vi "route_Ver.2.0.vi"(8 "error in (no error)":errorcluster, 9 "Position":T2, 11 "?":T1) -> (0 "error out":errorcluster, 1 "Position out":T2)   [LabVIEW 2019]
uses:
  subVI/move/position cluster.ctl
  route_name.ctl
  subVI/move control/move and align/move_cluster.ctl
  align position.ctl
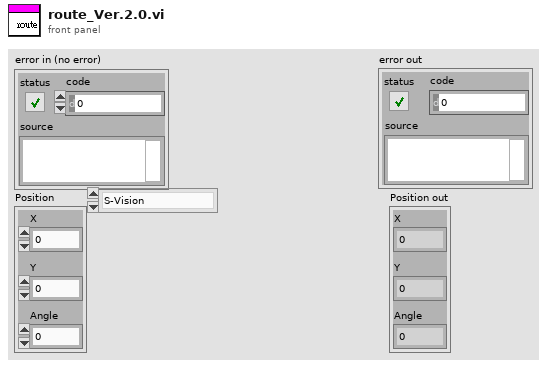
[diagram p1: front panel]
types:
  T1 = typedef "route_name.ctl" = enum16{"S-Vision", "Vision-R1", "Vision-R2", "Vision-R3", "Vision-R4", "Vision-R5", "R1-Vision", "R2-Vision", "R3-Vision", "R4-Vision", "R5-Vision", "Vision-box", "box-recycle", "recycle-box", "box-Vision", "Vision-S", "R2-R3"}
  T2 = typedef "position cluster.ctl" = cluster{"X":dbl, "Y":dbl, "Angle":dbl}
  T3 = typedef "move_cluster.ctl" = cluster{"X":dbl, "Y":dbl, "degree":dbl, "speed":dbl}
  T4 = typedef "align position.ctl" = enum16{"S align", "vision align", "box align", "box to room align"}
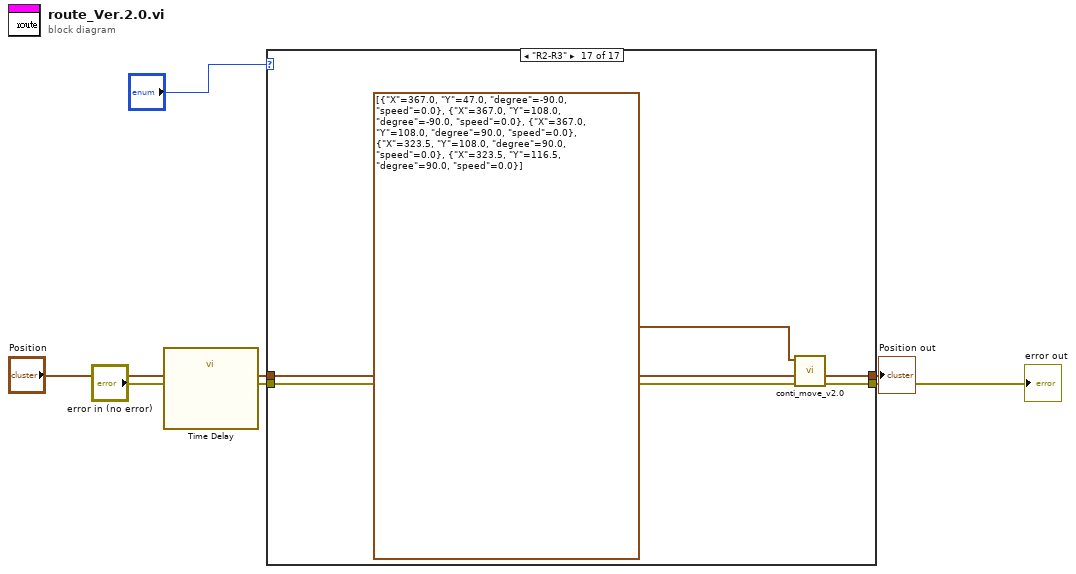
[diagram p0: block diagram]
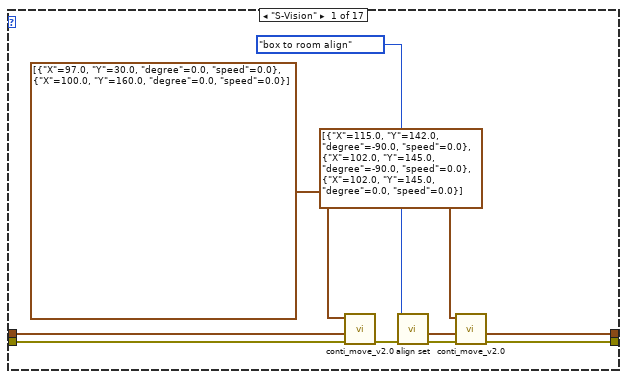
[diagram p2: hidden frame]
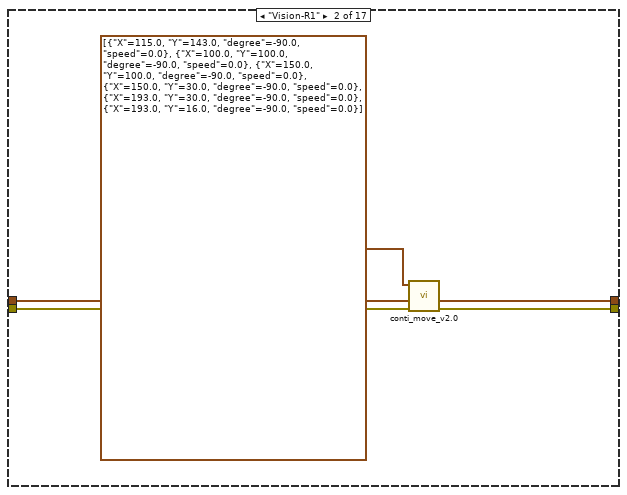
[diagram p3: hidden frame]
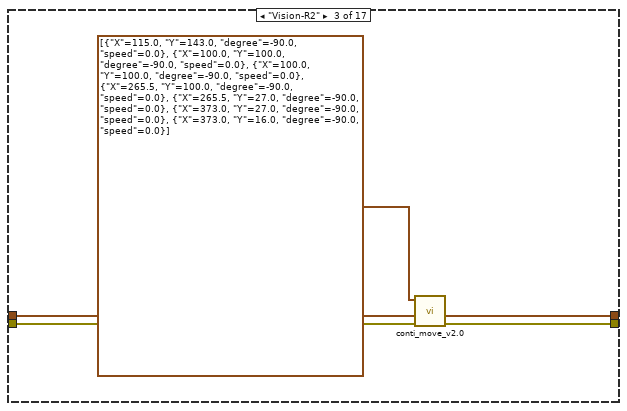
[diagram p4: hidden frame]
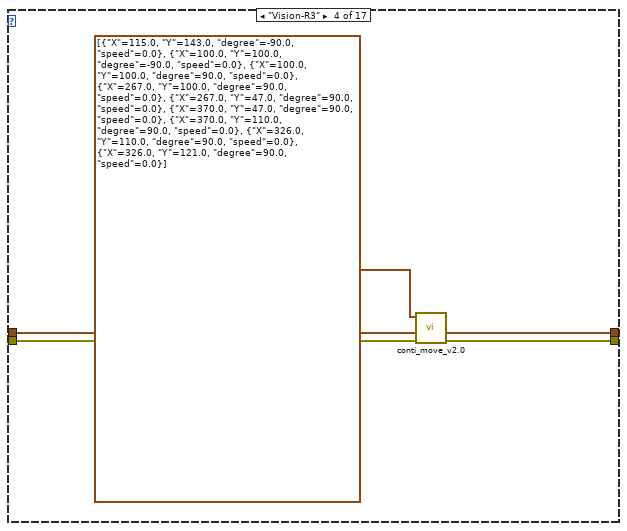
[diagram p5: hidden frame]
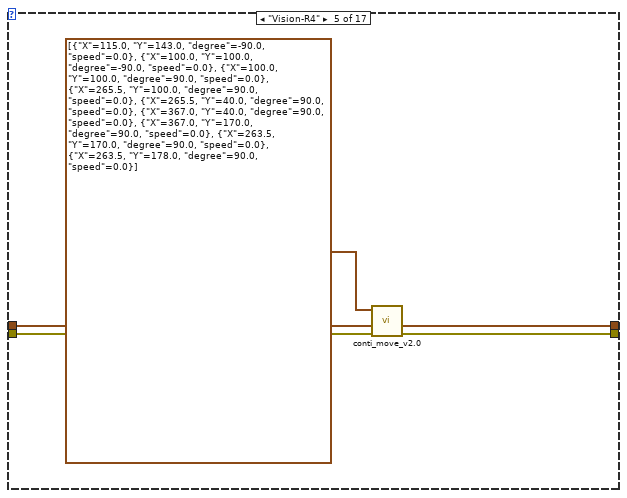
[diagram p6: hidden frame]
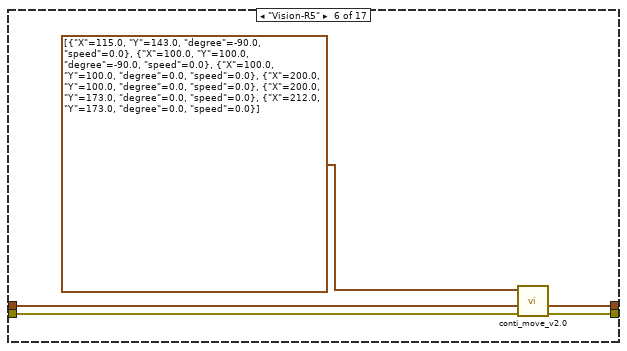
[diagram p7: hidden frame]
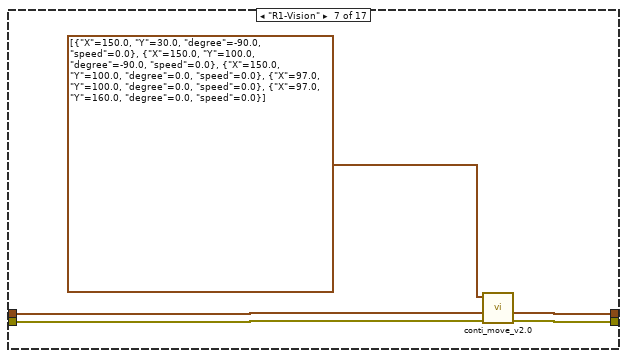
[diagram p8: hidden frame]
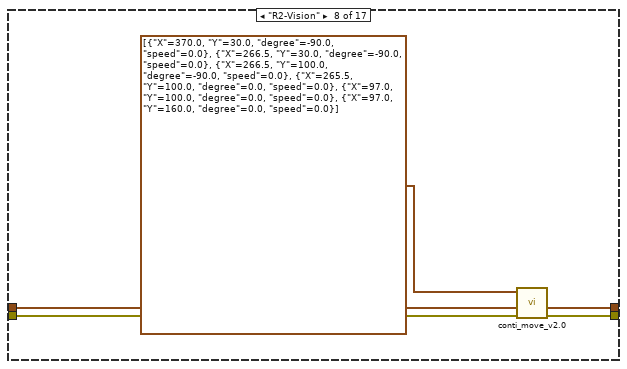
[diagram p9: hidden frame]
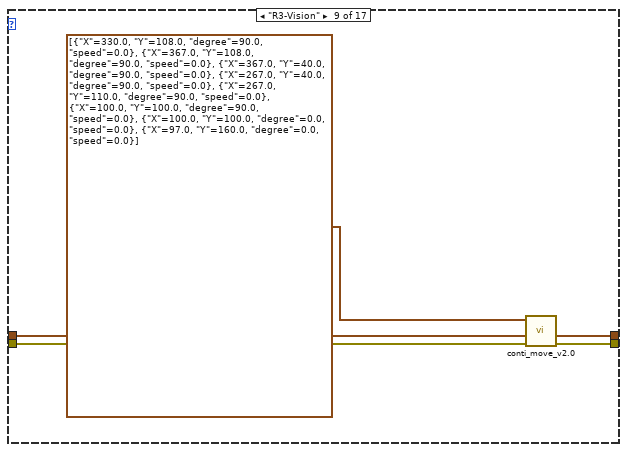
[diagram p10: hidden frame]
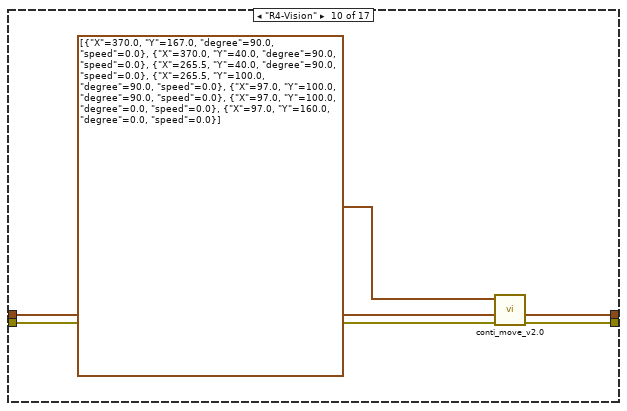
[diagram p11: hidden frame]
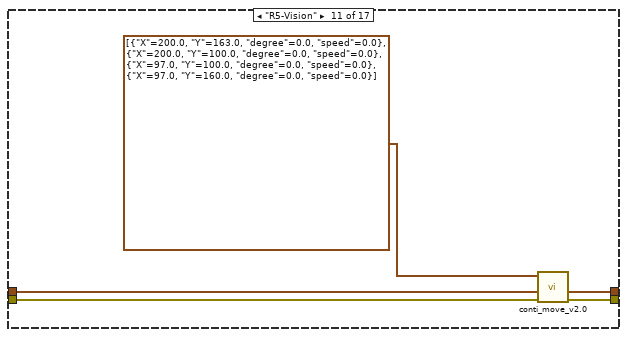
[diagram p12: hidden frame]
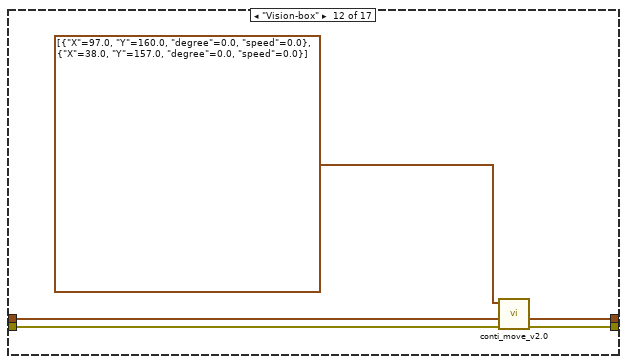
[diagram p13: hidden frame]
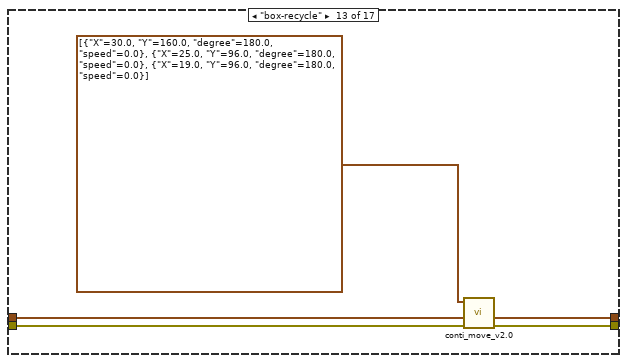
[diagram p14: hidden frame]
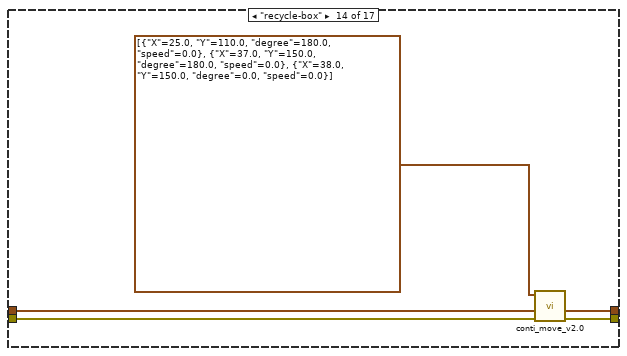
[diagram p15: hidden frame]
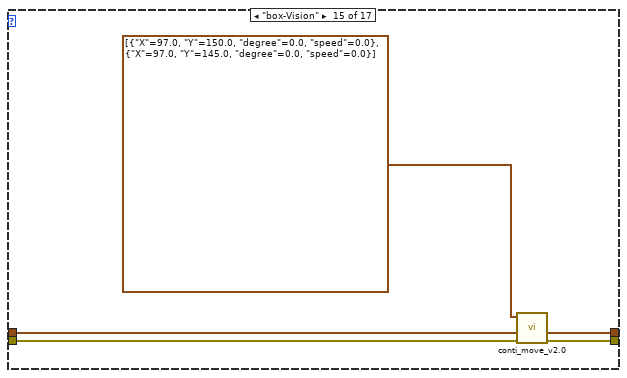
[diagram p16: hidden frame]
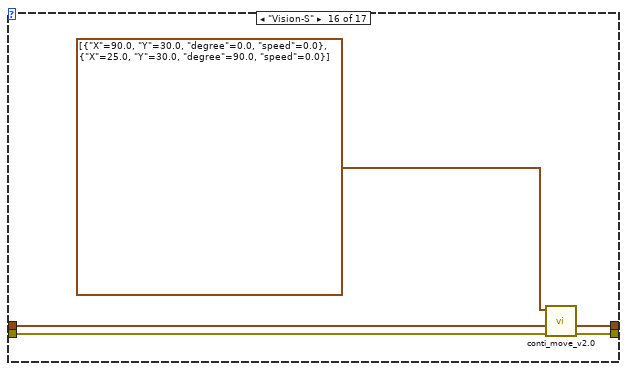
[diagram p17: hidden frame]
diagram:
  n1 = call "Time Delay"("error in (no error)"="error in (no error)") -> ("error out"=w1:errorcluster)  [unwired: 10 in]
  n2 = case shown="\"R2-R3\"" "?" {
    tunnel: w1 -> [w16 w20 w24 w27 w33 w39 w43 w49 w53 w59 w64 w69 w72 w78 w82 w88 w93]
    tunnel: "Position" -> [w15 w21 w25 w28 w34 w38 w44 w48 w54 w58 w63 w68 w74 w79 w83 w89 w94]
    tunnel: [w7 w19 w23 w30 w36 w41 w46 w51 w56 w61 w66 w71 w76 w81 w84 w91 w96] -> w3
    tunnel: [w8 w18 w22 w31 w35 w40 w45 w50 w55 w60 w65 w70 w75 w80 w85 w90 w95] -> w2
    frame "S-Vision" {
      n3 = call "conti_move_v2.0.vi"("error in (no error)"=w16, "Position"=w15, "route"=T3[] [{"X"=97.0, "Y"=30.0, "degree"=0.0, "speed"=0.0}, {"X"=100.0, "Y"=160.0, "degree"=0.0, "speed"=0.0}]) -> ("error out"=w13:errorcluster)  [unwired: 7 in, 1 out]
      n4 = call "align set.vi"("error in (no error)"=w13, "align position"=align_position."box to room align") -> ("error out"=w11:errorcluster, "position out"=w10:cluster{"X":dbl, "y":dbl, "degree":dbl})  [unwired: 8 in]
      n5 = call "conti_move_v2.0.vi"("error in (no error)"=w11, "Position"=w10, "route"=T3[] [{"X"=115.0, "Y"=142.0, "degree"=-90.0, "speed"=0.0}, {"X"=102.0, "Y"=145.0, "degree"=-90.0, "speed"=0.0}, {"X"=102.0, "Y"=145.0, "degree"=0.0, "speed"=0.0}] ("Array")) -> ("error out"=w7:errorcluster, "Position out"=w8:T2)  [unwired: 7 in]
    }
    frame "Vision-R1" {
      n6 = call "conti_move_v2.0.vi"("error in (no error)"=w20, "Position"=w21, "route"=T3[] [{"X"=115.0, "Y"=143.0, "degree"=-90.0, "speed"=0.0}, {"X"=100.0, "Y"=100.0, "degree"=-90.0, "speed"=0.0}, {"X"=150.0, "Y"=100.0, "degree"=-90.0, "speed"=0.0}, {"X"=150.0, "Y"=30.0, "degree"=-90.0, "speed"=0.0}, {"X"=193.0, "Y"=30.0, "degree"=-90.0, "speed"=0.0}, {"X"=193.0, "Y"=16.0, "degree"=-90.0, "speed"=0.0}]) -> ("error out"=w19:errorcluster, "Position out"=w18:T2)  [unwired: 7 in]
    }
    frame "Vision-R2" {
      n7 = call "conti_move_v2.0.vi"("error in (no error)"=w24, "Position"=w25, "route"=T3[] [{"X"=115.0, "Y"=143.0, "degree"=-90.0, "speed"=0.0}, {"X"=100.0, "Y"=100.0, "degree"=-90.0, "speed"=0.0}, {"X"=100.0, "Y"=100.0, "degree"=-90.0, "speed"=0.0}, {"X"=265.5, "Y"=100.0, "degree"=-90.0, "speed"=0.0}, {"X"=265.5, "Y"=27.0, "degree"=-90.0, "speed"=0.0}, {"X"=373.0, "Y"=27.0, "degree"=-90.0, "speed"=0.0}, {"X"=373.0, "Y"=16.0, "degree"=-90.0, "speed"=0.0}]) -> ("error out"=w23:errorcluster, "Position out"=w22:T2)  [unwired: 7 in]
    }
    frame "Vision-R3" {
      n8 = call "conti_move_v2.0.vi"("error in (no error)"=w27, "Position"=w28, "route"=T3[] [{"X"=115.0, "Y"=143.0, "degree"=-90.0, "speed"=0.0}, {"X"=100.0, "Y"=100.0, "degree"=-90.0, "speed"=0.0}, {"X"=100.0, "Y"=100.0, "degree"=90.0, "speed"=0.0}, {"X"=267.0, "Y"=100.0, "degree"=90.0, "speed"=0.0}, {"X"=267.0, "Y"=47.0, "degree"=90.0, "speed"=0.0}, {"X"=370.0, "Y"=47.0, "degree"=90.0, "speed"=0.0}, {"X"=370.0, "Y"=110.0, "degree"=90.0, "speed"=0.0}, {"X"=326.0, "Y"=110.0, "degree"=90.0, "speed"=0.0}, {"X"=326.0, "Y"=121.0, "degree"=90.0, "speed"=0.0}]) -> ("error out"=w30:errorcluster, "Position out"=w31:T2)  [unwired: 7 in]
    }
    frame "Vision-R4" {
      n9 = call "conti_move_v2.0.vi"("error in (no error)"=w33, "Position"=w34, "route"=T3[] [{"X"=115.0, "Y"=143.0, "degree"=-90.0, "speed"=0.0}, {"X"=100.0, "Y"=100.0, "degree"=-90.0, "speed"=0.0}, {"X"=100.0, "Y"=100.0, "degree"=90.0, "speed"=0.0}, {"X"=265.5, "Y"=100.0, "degree"=90.0, "speed"=0.0}, {"X"=265.5, "Y"=40.0, "degree"=90.0, "speed"=0.0}, {"X"=367.0, "Y"=40.0, "degree"=90.0, "speed"=0.0}, {"X"=367.0, "Y"=170.0, "degree"=90.0, "speed"=0.0}, {"X"=263.5, "Y"=170.0, "degree"=90.0, "speed"=0.0}, {"X"=263.5, "Y"=178.0, "degree"=90.0, "speed"=0.0}]) -> ("error out"=w36:errorcluster, "Position out"=w35:T2)  [unwired: 7 in]
    }
    frame "Vision-R5" {
      n10 = call "conti_move_v2.0.vi"("error in (no error)"=w39, "Position"=w38, "route"=T3[] [{"X"=115.0, "Y"=143.0, "degree"=-90.0, "speed"=0.0}, {"X"=100.0, "Y"=100.0, "degree"=-90.0, "speed"=0.0}, {"X"=100.0, "Y"=100.0, "degree"=0.0, "speed"=0.0}, {"X"=200.0, "Y"=100.0, "degree"=0.0, "speed"=0.0}, {"X"=200.0, "Y"=173.0, "degree"=0.0, "speed"=0.0}, {"X"=212.0, "Y"=173.0, "degree"=0.0, "speed"=0.0}]) -> ("error out"=w41:errorcluster, "Position out"=w40:T2)  [unwired: 7 in]
    }
    frame "R1-Vision" {
      n11 = call "conti_move_v2.0.vi"("error in (no error)"=w43, "Position"=w44, "route"=T3[] [{"X"=150.0, "Y"=30.0, "degree"=-90.0, "speed"=0.0}, {"X"=150.0, "Y"=100.0, "degree"=-90.0, "speed"=0.0}, {"X"=150.0, "Y"=100.0, "degree"=0.0, "speed"=0.0}, {"X"=97.0, "Y"=100.0, "degree"=0.0, "speed"=0.0}, {"X"=97.0, "Y"=160.0, "degree"=0.0, "speed"=0.0}]) -> ("error out"=w46:errorcluster, "Position out"=w45:T2)  [unwired: 7 in]
    }
    frame "R2-Vision" {
      n12 = call "conti_move_v2.0.vi"("error in (no error)"=w49, "Position"=w48, "route"=T3[] [{"X"=370.0, "Y"=30.0, "degree"=-90.0, "speed"=0.0}, {"X"=266.5, "Y"=30.0, "degree"=-90.0, "speed"=0.0}, {"X"=266.5, "Y"=100.0, "degree"=-90.0, "speed"=0.0}, {"X"=265.5, "Y"=100.0, "degree"=0.0, "speed"=0.0}, {"X"=97.0, "Y"=100.0, "degree"=0.0, "speed"=0.0}, {"X"=97.0, "Y"=160.0, "degree"=0.0, "speed"=0.0}]) -> ("error out"=w51:errorcluster, "Position out"=w50:T2)  [unwired: 7 in]
    }
    frame "R3-Vision" {
      n13 = call "conti_move_v2.0.vi"("error in (no error)"=w53, "Position"=w54, "route"=T3[] [{"X"=330.0, "Y"=108.0, "degree"=90.0, "speed"=0.0}, {"X"=367.0, "Y"=108.0, "degree"=90.0, "speed"=0.0}, {"X"=367.0, "Y"=40.0, "degree"=90.0, "speed"=0.0}, {"X"=267.0, "Y"=40.0, "degree"=90.0, "speed"=0.0}, {"X"=267.0, "Y"=110.0, "degree"=90.0, "speed"=0.0}, {"X"=100.0, "Y"=100.0, "degree"=90.0, "speed"=0.0}, {"X"=100.0, "Y"=100.0, "degree"=0.0, "speed"=0.0}, {"X"=97.0, "Y"=160.0, "degree"=0.0, "speed"=0.0}]) -> ("error out"=w56:errorcluster, "Position out"=w55:T2)  [unwired: 7 in]
    }
    frame "R4-Vision" {
      n14 = call "conti_move_v2.0.vi"("error in (no error)"=w59, "Position"=w58, "route"=T3[] [{"X"=370.0, "Y"=167.0, "degree"=90.0, "speed"=0.0}, {"X"=370.0, "Y"=40.0, "degree"=90.0, "speed"=0.0}, {"X"=265.5, "Y"=40.0, "degree"=90.0, "speed"=0.0}, {"X"=265.5, "Y"=100.0, "degree"=90.0, "speed"=0.0}, {"X"=97.0, "Y"=100.0, "degree"=90.0, "speed"=0.0}, {"X"=97.0, "Y"=100.0, "degree"=0.0, "speed"=0.0}, {"X"=97.0, "Y"=160.0, "degree"=0.0, "speed"=0.0}]) -> ("error out"=w61:errorcluster, "Position out"=w60:T2)  [unwired: 7 in]
    }
    frame "R5-Vision" {
      n15 = call "conti_move_v2.0.vi"("error in (no error)"=w64, "Position"=w63, "route"=T3[] [{"X"=200.0, "Y"=163.0, "degree"=0.0, "speed"=0.0}, {"X"=200.0, "Y"=100.0, "degree"=0.0, "speed"=0.0}, {"X"=97.0, "Y"=100.0, "degree"=0.0, "speed"=0.0}, {"X"=97.0, "Y"=160.0, "degree"=0.0, "speed"=0.0}]) -> ("error out"=w66:errorcluster, "Position out"=w65:T2)  [unwired: 7 in]
    }
    frame "Vision-box" {
      n16 = call "conti_move_v2.0.vi"("error in (no error)"=w69, "Position"=w68, "route"=T3[] [{"X"=97.0, "Y"=160.0, "degree"=0.0, "speed"=0.0}, {"X"=38.0, "Y"=157.0, "degree"=0.0, "speed"=0.0}]) -> ("error out"=w71:errorcluster, "Position out"=w70:T2)  [unwired: 7 in]
    }
    frame "box-recycle" {
      n17 = call "conti_move_v2.0.vi"("error in (no error)"=w72, "Position"=w74, "route"=T3[] [{"X"=30.0, "Y"=160.0, "degree"=180.0, "speed"=0.0}, {"X"=25.0, "Y"=96.0, "degree"=180.0, "speed"=0.0}, {"X"=19.0, "Y"=96.0, "degree"=180.0, "speed"=0.0}]) -> ("error out"=w76:errorcluster, "Position out"=w75:T2)  [unwired: 7 in]
    }
    frame "recycle-box" {
      n18 = call "conti_move_v2.0.vi"("error in (no error)"=w78, "Position"=w79, "route"=T3[] [{"X"=25.0, "Y"=110.0, "degree"=180.0, "speed"=0.0}, {"X"=37.0, "Y"=150.0, "degree"=180.0, "speed"=0.0}, {"X"=38.0, "Y"=150.0, "degree"=0.0, "speed"=0.0}]) -> ("error out"=w81:errorcluster, "Position out"=w80:T2)  [unwired: 7 in]
    }
    frame "box-Vision" {
      n19 = call "conti_move_v2.0.vi"("error in (no error)"=w82, "Position"=w83, "route"=T3[] [{"X"=97.0, "Y"=150.0, "degree"=0.0, "speed"=0.0}, {"X"=97.0, "Y"=145.0, "degree"=0.0, "speed"=0.0}]) -> ("error out"=w84:errorcluster, "Position out"=w85:T2)  [unwired: 7 in]
    }
    frame "Vision-S" {
      n20 = call "conti_move_v2.0.vi"("error in (no error)"=w88, "Position"=w89, "route"=T3[] [{"X"=90.0, "Y"=30.0, "degree"=0.0, "speed"=0.0}, {"X"=25.0, "Y"=30.0, "degree"=90.0, "speed"=0.0}]) -> ("error out"=w91:errorcluster, "Position out"=w90:T2)  [unwired: 7 in]
    }
    frame "R2-R3" {
      n21 = call "conti_move_v2.0.vi"("error in (no error)"=w93, "Position"=w94, "route"=T3[] [{"X"=367.0, "Y"=47.0, "degree"=-90.0, "speed"=0.0}, {"X"=367.0, "Y"=108.0, "degree"=-90.0, "speed"=0.0}, {"X"=367.0, "Y"=108.0, "degree"=90.0, "speed"=0.0}, {"X"=323.5, "Y"=108.0, "degree"=90.0, "speed"=0.0}, {"X"=323.5, "Y"=116.5, "degree"=90.0, "speed"=0.0}]) -> ("error out"=w96:errorcluster, "Position out"=w95:T2)  [unwired: 7 in]
    }
  }
  "error out" <- w3
  "Position out" <- w2
